vi "Send.vi"(8 "error in (no error)":errorcluster, 9 "Data":string, 10 "Client ID":string, 11 "WebSocket Service Actor in":refnum<class "WebSocket Service.lvclass">) -> (0 "error out":errorcluster, 3 "WebSocket Service Actor out":refnum<class "WebSocket Service.lvclass">)   [LabVIEW 2021, in "WebSocket Actors.lvlib" / "WebSocket Service.lvclass"]
doc: "Sends data to the client identified by Client ID"
uses:
  WebSocket Service.lvclass
  WebSocket Service.lvclass/WebSocket Service.ctl
  <vilib>/ActorFramework/Message Enqueuer/Message Enqueuer.lvclass
  WebSocket Connection Messages/Send to Peer Msg/Send to Peer Msg.lvclass
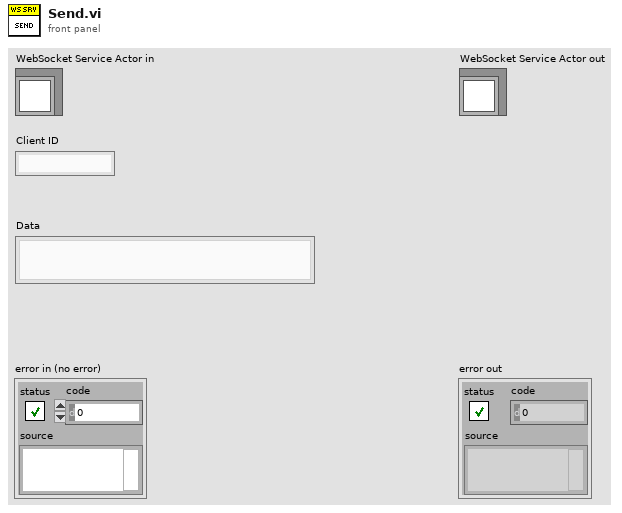
[diagram p1: front panel]
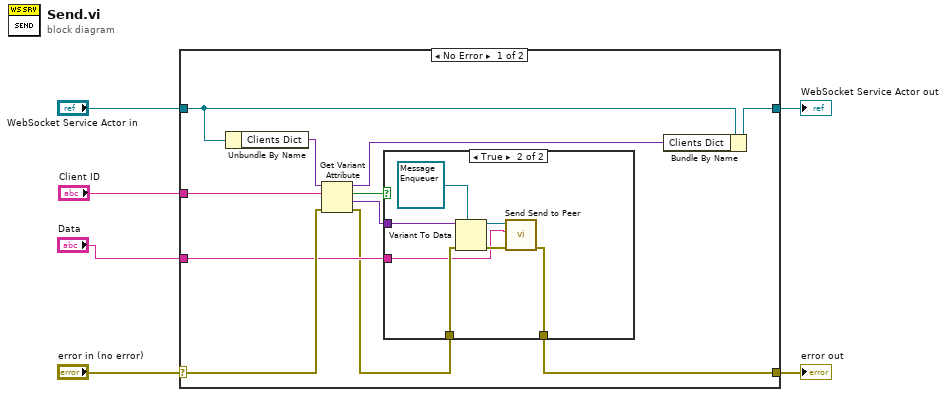
[diagram p0: block diagram]
diagram:
  n1 = case shown="No Error" "error in (no error)" {
    selector: "error in (no error)" -> [w13 w27]
    tunnel: [w7 w27] -> w5
    tunnel: [w16 w26] -> w3
    tunnel: "WebSocket Service Actor in" -> [w17 w26]
    tunnel: "Client ID" -> [w15 _]
    tunnel: "Data" -> [w9 _]
    frame No Error {
      n2 = Unbundle By Name(w17) -> ("Clients Dict"=w14:variant)
      n3 = Get Variant Attribute(Variant=w14, name=w15, error in=w13) -> (duplicate Variant=w11:variant, found=w12:bool, value=w10:variant, error out=w8:errorcluster)  [unwired: 1 in]
      n4 = case shown="True" w12 {
        tunnel: w10 -> [_ w24]
        tunnel: w8 -> [w18 w23]
        tunnel: w9 -> [_ w21]
        tunnel: [w18 w19] -> w7
        frame False {
        }
        frame True {
          n5 = Variant To Data(error in=w23, type=refnum<class "Message Enqueuer.lvclass"> refnum ("Message Enqueuer in"), Variant=w24) -> (data=w20:refnum<class "Message Enqueuer.lvclass">, error out=w22:errorcluster)
          n6 = call "Send Send to Peer.vi"("error in (no error)"=w22, "Data"=w21, "Message Enqueuer in"=w20) -> ("error out"=w19:errorcluster)  [unwired: 7 in, 1 out]
        }
      }
      n7 = Bundle By Name(cluster=w17, "Clients Dict"=w11) -> (w16:refnum<class "WebSocket Service.lvclass">)
    }
    frame Error {
    }
  }
  "error out" <- w5
  "WebSocket Service Actor out" <- w3
